vi "Calculate Encapsulant Cureness.vi"(10 "Mixing Time":timestamp, 11 "Potting Parameters":T1) -> (3 "Cureness":dbl)   [LabVIEW 2011]
uses:
  Config Manager Class/Type Definitions/Potting Parameters.ctl
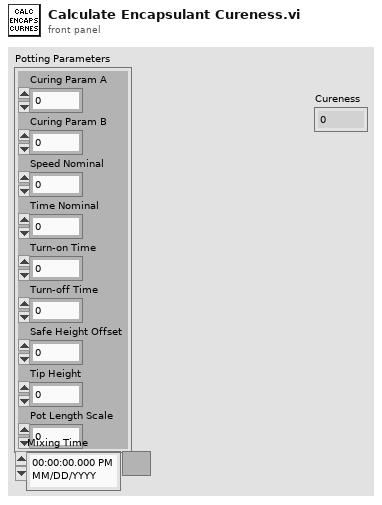
[diagram p1: front panel]
types:
  T1 = typedef "Potting Parameters.ctl" = cluster{"Curing Param A":dbl, "Curing Param B":dbl, "Speed Nominal":dbl, "Time Nominal":dbl, "Turn-on Time":dbl, "Turn-off Time":dbl, "Safe Height Offset":dbl, "Tip Height":dbl, "Pot Length Scale":dbl}
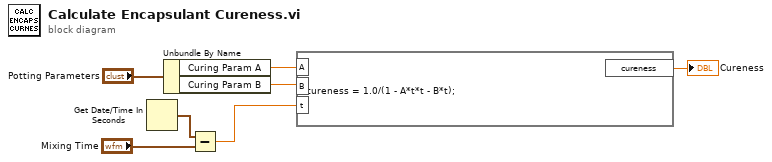
[diagram p0: block diagram]
diagram:
  n1 = Get Date/Time In Seconds() -> (seconds since 1Jan1904=w5:timestamp)
  n2 = Unbundle By Name("Potting Parameters") -> ("Curing Param A"=w4:dbl, "Curing Param B"=w3:dbl)
  n3 = Subtract(x=w5, y="Mixing Time") -> (x-y=w2:dbl)
  n4 = formula code="cureness = 1.0/(1 - A*t*t - B*t);"("A"=w4, "B"=w3, "t"=w2) -> ("cureness"=→"Cureness":dbl)
